vi "GetViRootPath.vi"(1 "VI引用句柄":refnum<vi>) -> (0 "RootPath":path)   [LabVIEW 2012]
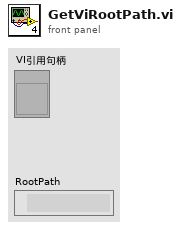
[diagram p1: front panel]
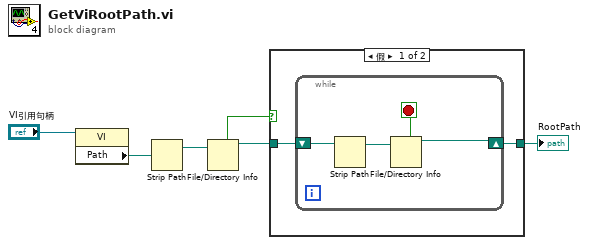
[diagram p0: block diagram]
diagram:
  n1 = property class="VI"(reference="VI引用句柄") -> ("Path"=w5:path)  [unwired: 1 in, 2 out]
  n2 = Strip Path(path=w5) -> (stripped path=w4:path)  [unwired: 1 out]
  n3 = File/Directory Info(path=w4) -> (path out=w2:path, directory=w3:bool)  [unwired: 1 in, 5 out]
  n4 = case shown="假" w3 {
    tunnel: [w7 w13] -> w1
    tunnel: w2 -> [w8 w13]
    frame False {
      n5 = while {
        shift-right: [w9] -> w7
        shift-left: w8 -> [w12]
        stop <- w10 stop-if-true
        n6 = Strip Path(path=w12) -> (stripped path=w11:path)  [unwired: 1 out]
        n7 = File/Directory Info(path=w11) -> (path out=w9:path, directory=w10:bool)  [unwired: 1 in, 5 out]
      }
    }
    frame True {
    }
  }
  "RootPath" <- w1
